vi "Graph_FPGA_stripped_v00.vi"() -> ()   [LabVIEW 2010]
uses:
  Strict Type Defs/Graph Errors.ctl
  Strict Type Defs/Graph Lock Point.ctl
  Strict Type Defs/Graph Output.ctl
  Strict Type Defs/Control Graph Input.ctl
  Strict Type Defs/PII individual.ctl
  Strict Type Defs/Error Scale Graph.ctl
  Strict Type Defs/Lock Thresh Graph.ctl
  Strict Type Defs/Theta graph.ctl
  Strict Type Defs/Safety First.ctl
  Strict Type Defs/Scope.ctl
  Strict Type Defs/Graph Max.ctl
  Strict Type Defs/Graph Min.ctl
  <vilib>/rvi/DataTransferAndStorage/Container/XNode/niFpgaContainer.xnode
  <vilib>/rvi/DataTransferAndStorage/Container/Common/niFpgaContainerMethod.ctl
  <vilib>/rvi/DataTransferAndStorage/Container/Common/niFpgaTransferTypeControl.ctl
  <vilib>/rvi/interface/RandomDataEmulation/nirviRandomDataFPGAFIFO.vi
  <vilib>/rvi/interface/RandomDataEmulation/niFpgaRandomDataHandleErrors.vi
panel:
  out "Min":T1
  out "Max":T2
  in  "Graph Delay(uSec)":u32 caption="Count(uSec)"
  out "HD Errors xp":T3
  in  "Scope":T4={"Trigger Direction"=enum."plus-minus", "Delay"=0, "Aquisition Rate (Ticks)"=40, "Offset"=0, "Channel"=0, "Channel Selector"={"Channel 1"=0, "Channel 2"=4, "Channel 3"=8, "Channel 4"=8}} {"Channel Selector"."Channel 4" items=["Error Signal 1", "Error Signal 2", "Scan Trigger 1", "Scan Trigger 2", "DC Signal 1", "DC Signal 2", "PI Out 1", "PI Out 2"]; "Channel Selector"."Channel 3" items=["Error Signal 1", "Error Signal 2", "Scan Trigger 1", "Scan Trigger 2", "DC Signal 1", "DC Signal 2", "PI Out 1", "PI Out 2"]; "Channel Selector"."Channel 2" items=["Error Signal 1", "Error Signal 2", "Scan Trigger 1", "Scan Trigger 2", "DC Signal 1", "DC Signal 2", "PI Out 1", "PI Out 2"]; "Channel Selector"."Channel 1" items=["Error Signal 1", "Error Signal 2", "Scan Trigger 1", "Scan Trigger 2", "DC Signal 1", "DC Signal 2", "PI Out 1", "PI Out 2"]}
  in  "quit Control Loop":bool
  in  "Control":T5={"PII In 1"={"Lock"=FALSE, "Hold"=FALSE, "P Gain"=0, "P BS"=-5, "I Gain"=0, "I BS"=-10, "I2 G"=0, "I2 BS"=-26, "Scan Amp"=0, "Scan Off"=0, "Scan FS"=0, "SFS BS"=0, "I Max value"=10000, "I2 Max value"=10000, "Scope.Offset"=0, "Trigger Direction"=enum."either", "Scan-PII thresh"=0}, "PII In 2"={"Lock"=FALSE, "Hold"=FALSE, "P Gain"=0, "P BS"=-10, "I Gain"=0, "I BS"=-10, "I2 G"=0, "I2 BS"=-26, "Scan Amp"=0, "Scan Off"=0, "Scan FS"=0, "SFS BS"=0, "I Max value"=10000, "I2 Max value"=10000, "Scope.Offset"=0, "Trigger Direction"=enum."either", "Scan-PII thresh"=0}, "PII In 3"={"Lock"=FALSE, "Hold"=FALSE, "P Gain"=0, "P BS"=-10, "I Gain"=0, "I BS"=-10, "I2 G"=0, "I2 BS"=-26, "Scan Amp"=0, "Scan Off"=0, "Scan FS"=0, "SFS BS"=0, "I Max value"=10000, "I2 Max value"=10000, "Scope.Offset"=0, "Trigger Direction"=enum."either", "Scan-PII thresh"=0}, "PII In 4"={"Lock"=FALSE, "Hold"=FALSE, "P Gain"=0, "P BS"=-10, "I Gain"=0, "I BS"=-10, "I2 G"=0, "I2 BS"=-26, "Scan Amp"=0, "Scan Off"=0, "Scan FS"=0, "SFS BS"=0, "I Max value"=10000, "I2 Max value"=10000, "Scope.Offset"=0, "Trigger Direction"=enum."either", "Scan-PII thresh"=0}, "PII In 5"={"Lock"=FALSE, "Hold"=FALSE, "P Gain"=10, "P BS"=-10, "I Gain"=0, "I BS"=0, "I2 G"=0, "I2 BS"=-26, "Scan Amp"=0, "Scan Off"=0, "Scan FS"=0, "SFS BS"=0, "I Max value"=10000, "I2 Max value"=10000, "Scope.Offset"=0, "Trigger Direction"=enum."either", "Scan-PII thresh"=0}, "PII In 6"={"Lock"=FALSE, "Hold"=FALSE, "P Gain"=0, "P BS"=-10, "I Gain"=0, "I BS"=-10, "I2 G"=0, "I2 BS"=-26, "Scan Amp"=0, "Scan Off"=0, "Scan FS"=0, "SFS BS"=0, "I Max value"=10000, "I2 Max value"=10000, "Scope.Offset"=0, "Trigger Direction"=enum."either", "Scan-PII thresh"=0}, "Error scale"={"Pre-Offset"={"Pre-Offset 1"=2, "Pre-Offset 2"=0, "Pre-Offset 3"=0, "Pre-Offset 4"=0, "Pre-Offset 5"=2, "Pre-Offset 6"=0, "Pre-Offset 7"=0, "Pre-Offset 8"=0}, "Post-Offset "={"Offset 1"=0, "Offset 2"=300, "Offset 3"=0, "Offset 4"=0, "Offset 5"=0, "Offset 6"=0, "Offset 7"=0, "Offset 8"=0}, "Gains"={"Gain 1"=0, "Gain 2"=300, "Gain 3"=0, "Gain 4"=0, "Gain 5"=0, "Gain 6"=0, "Gain 7"=0, "Gain 8"=0}, "Bit Shifts"={"Bit Shift 1"=0, "Bit Shift 2"=300, "Bit Shift 3"=0, "Bit Shift 4"=0, "Bit Shift 5"=0, "Bit Shift 6"=0, "Bit Shift 7"=0, "Bit Shift 8"=0}}, "Lock Thresh"={"Pump A"=0, "Pump B"=0, "EPR"=0, "Graph"=0, "HD A"=40, "HD B"=0}, "Re-Scan Thresh"={"Pump A"=2, "Pump B"=0, "EPR"=40, "Graph"=0, "HD A"=40, "HD B"=0}, "Theta"={"HD A Sin Theta"=0, "HD A Cos Theta"=0, "HD B Sin Theta"=0, "HD B Cos Theta"=0}, "Safety First"={"lim reset"=FALSE, "no limit"=FALSE, "pos slew rate * dt"=10, "neg slew rate * dt"=-10, "Hold All"=FALSE, "Count(Ticks)"=0}}
  in  "\"I too high?\"":T11
  in  "\"Outputs\"":T12
  out "Outputs":T12={"Pump A"=-270, "Pump B"=-1710, "EPR"=880, "Graph"=570, "HD A"=0, "HD B"=0}
  in  "\"Trigger\"":T11
  out "Trigger":T11
  out "Cavity Errors":T13={"Pump A"=0, "Pump B"=1800, "EPR"=0, "Graph"=0, "HD A"=0, "HD B"=0}
  out "Control Loop count":i32=11285327
  out "Scope Full?":bool
  out "Scope loop count":i32=119818
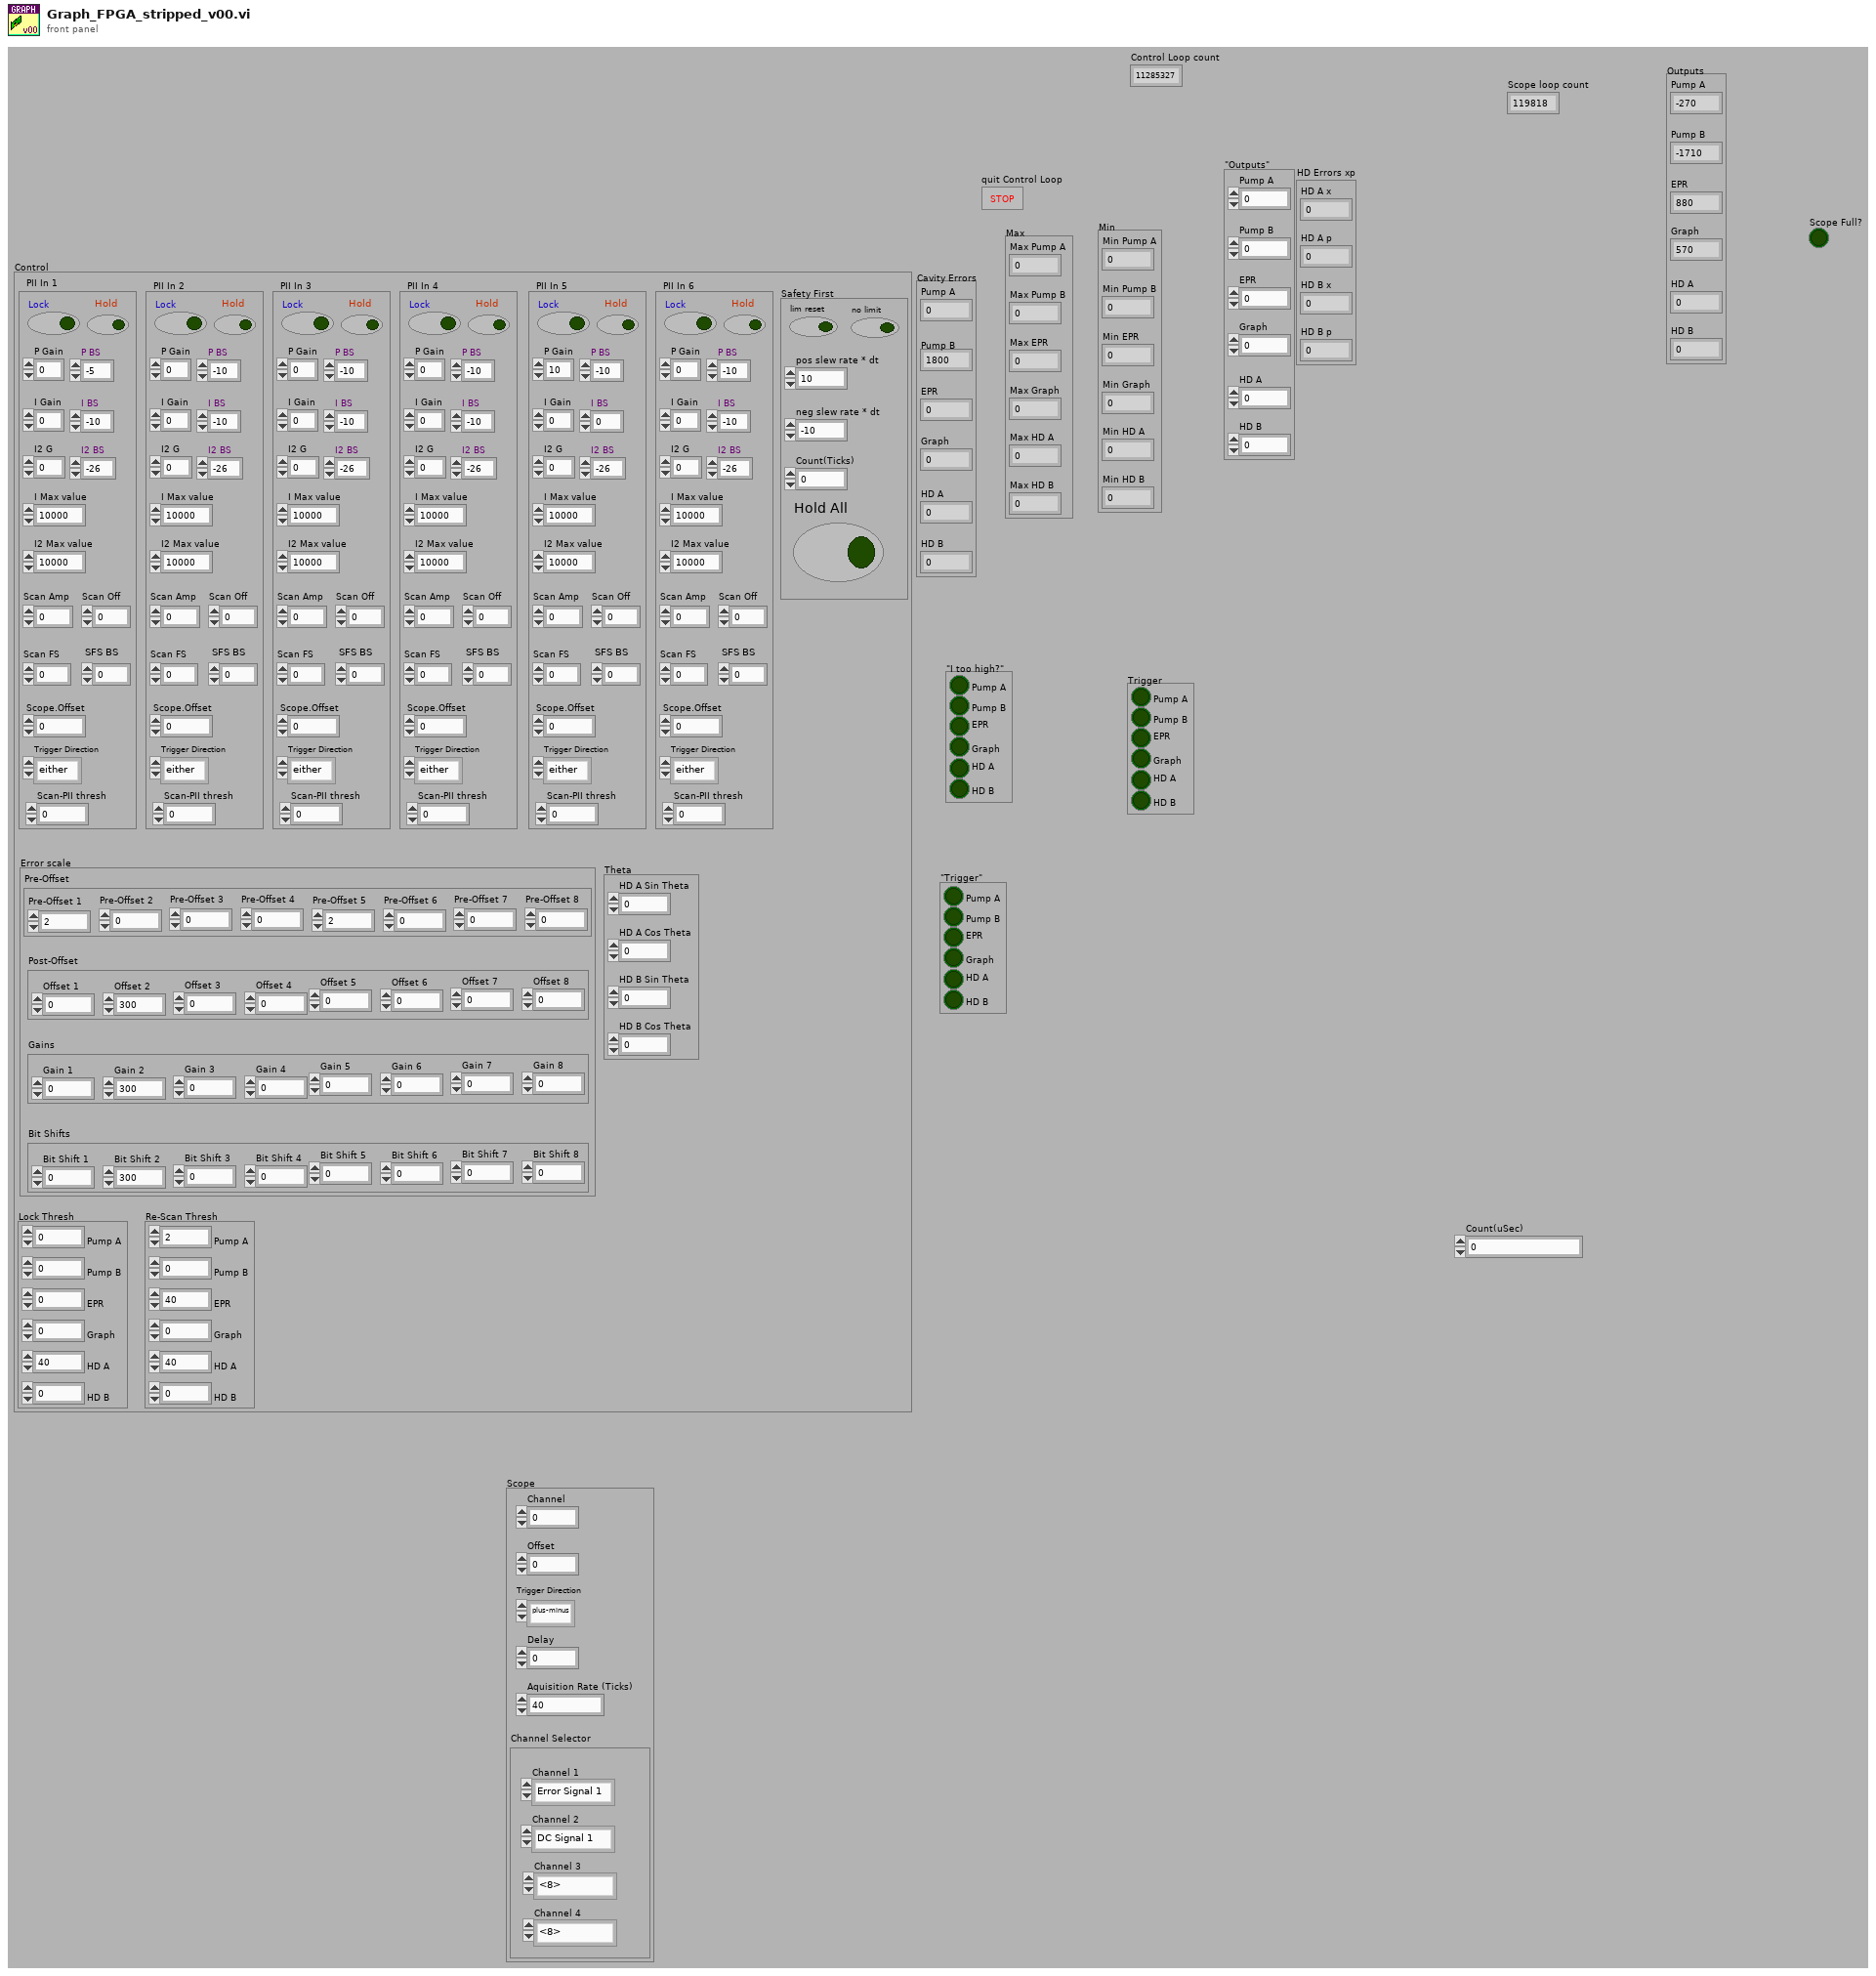
[diagram p1: front panel]
types:
  T1 = typedef "Graph Min.ctl" = cluster{"Min Pump A":i16, "Min Pump B":i16, "Min EPR":i16, "Min Graph":i16, "Min HD A":i16, "Min HD B":i16}
  T2 = typedef "Graph Max.ctl" = cluster{"Max Pump A":i16, "Max Pump B":i16, "Max EPR":i16, "Max Graph":i16, "Max HD A":i16, "Max HD B":i16}
  T3 = cluster{"HD A x":i16, "HD A p":i16, "HD B x":i16, "HD B p":i16}
  T4 = typedef "Scope.ctl" = cluster{"Trigger Direction":enum8{"either", "minus-plus", "plus-minus"}, "Delay":u32, "Aquisition Rate (Ticks)":u32, "Offset":i16, "Channel":i32, "Channel Selector":cluster{"Channel 1":i32, "Channel 2":i32, "Channel 3":i32, "Channel 4":i32}}
  T5 = typedef "Control Graph Input.ctl" = cluster{"PII In 1":T6, "PII In 2":T6, "PII In 3":T6, "PII In 4":T6, "PII In 5":T6, "PII In 6":T6, "Error scale":T7, "Lock Thresh":T8, "Re-Scan Thresh":T8, "Theta":T9, "Safety First":T10}
  T6 = typedef "PII individual.ctl" = cluster{"Lock":bool, "Hold":bool, "P Gain":i32, "P BS":i16, "I Gain":i32, "I BS":i16, "I2 G":i32, "I2 BS":i16, "Scan Amp":i16, "Scan Off":i16, "Scan FS":u16, "SFS BS":i16, "I Max value":i32, "I2 Max value":i32, "Scope.Offset":i16, "Trigger Direction":enum8{"either", "minus-plus", "plus-minus"}, "Scan-PII thresh":i16}
  T7 = typedef "Error Scale Graph.ctl" = cluster{"Pre-Offset":cluster{"Pre-Offset 1":i16, "Pre-Offset 2":i16, "Pre-Offset 3":i16, "Pre-Offset 4":i16, "Pre-Offset 5":i16, "Pre-Offset 6":i16, "Pre-Offset 7":i16, "Pre-Offset 8":i16}, "Post-Offset ":cluster{"Offset 1":i16, "Offset 2":i16, "Offset 3":i16, "Offset 4":i16, "Offset 5":i16, "Offset 6":i16, "Offset 7":i16, "Offset 8":i16}, "Gains":cluster{"Gain 1":i16, "Gain 2":i16, "Gain 3":i16, "Gain 4":i16, "Gain 5":i16, "Gain 6":i16, "Gain 7":i16, "Gain 8":i16}, "Bit Shifts":cluster{"Bit Shift 1":i16, "Bit Shift 2":i16, "Bit Shift 3":i16, "Bit Shift 4":i16, "Bit Shift 5":i16, "Bit Shift 6":i16, "Bit Shift 7":i16, "Bit Shift 8":i16}}
  T8 = typedef "Lock Thresh Graph.ctl" = cluster{"Pump A":i16, "Pump B":i16, "EPR":i16, "Graph":i16, "HD A":i16, "HD B":i16}
  T9 = typedef "Theta graph.ctl" = cluster{"HD A Sin Theta":i32, "HD A Cos Theta":i32, "HD B Sin Theta":i32, "HD B Cos Theta":i32}
  T10 = typedef "Safety First.ctl" = cluster{"lim reset":bool, "no limit":bool, "pos slew rate * dt":i16, "neg slew rate * dt":i16, "Hold All":bool, "Count(Ticks)":u32}
  T11 = typedef "Graph Lock Point.ctl" = cluster{"Pump A":bool, "Pump B":bool, "EPR":bool, "Graph":bool, "HD A":bool, "HD B":bool}
  T12 = typedef "Graph Output.ctl" = cluster{"Pump A":i16, "Pump B":i16, "EPR":i16, "Graph":i16, "HD A":i16, "HD B":i16}
  T13 = typedef "Graph Errors.ctl" = cluster{"Pump A":i16, "Pump B":i16, "EPR":i16, "Graph":i16, "HD A":i16, "HD B":i16}
  T14 = typedef "Signals Graph.ctl" = cluster{"PII In 1":T6, "PII In 2":T6, "PII In 3":T6, "PII In 4":T6, "PII In 5":T6, "PII In 6":T6, "Lock Thresh":T8, "Re-Scan Thresh":T8, "Safety First":T10, "Graph Errors":T13}
  T15 = typedef "Graph Control Cluster.ctl" = cluster{"Control Pump A":T6, "Control Pump B":T6, "Control EPR":T6, "Control Graph":T6, "Control HD A":T6, "Control HD B":T6, "Max":T2, "Min":T1, "Lock Threshold":T8, "Re-Scan Threshold":T8, "Lock Point?":T11, "Re-scan?":T11, "Lock pressed? (-1)":T11, "Cavity Errors":T13, "State (-1)":T16, "Safety First":T10}
  T16 = typedef "Graph State.ctl" = cluster{"Pump A":enum16{"Safe", "Hold", "Scan", "Lock"}, "Pump B":enum16{"Safe", "Hold", "Scan", "Lock"}, "EPR":enum16{"Safe", "Hold", "Scan", "Lock"}, "Graph":enum16{"Safe", "Hold", "Scan", "Lock"}, "HD A":enum16{"Safe", "Hold", "Scan", "Lock"}, "HD B":enum16{"Safe", "Hold", "Scan", "Lock"}}
  T17 = typedef "Graph PII Scan State.ctl" = cluster{"Control Pump A":T6, "Control Pump B":T6, "Control EPR":T6, "Control Graph":T6, "Control HD A":T6, "Control HD B":T6, "Error Signals":T13, "State":T16}
  T18 = typedef "Graph MaxMin.ctl" = cluster{"State":T16, "Reset MaxMin?":T19, "Max":T2, "Min":T1, "Lock pressed?":T11, "Safety First":T10}
  T19 = typedef "Graph Reset MaxMin.ctl" = cluster{"Pump A":bool, "Pump B":bool, "EPR":bool, "Graph":bool, "HD A":bool, "HD B":bool}
  T20 = typedef "niFpgaContainerMethod.ctl" = enum16{"<none>", "write", "read", "clear", "getNumberOfElementsToWrite", "getNumberOfElementsToRead", "enable", "disable", "flushAndDisable", "getStreamState", "readA", "readB", "dramWrite", "dramWriteWithByteEnables", "dramRequestData", "dramRetrieveData"}
  T21 = typedef "niFpgaTransferTypeControl.ctl" = enum16{"Target-Scoped", "Host to Target - DMA", "Target to Host - DMA", "Peer to Peer Reader", "Peer to Peer Writer", "Bidirectional"}
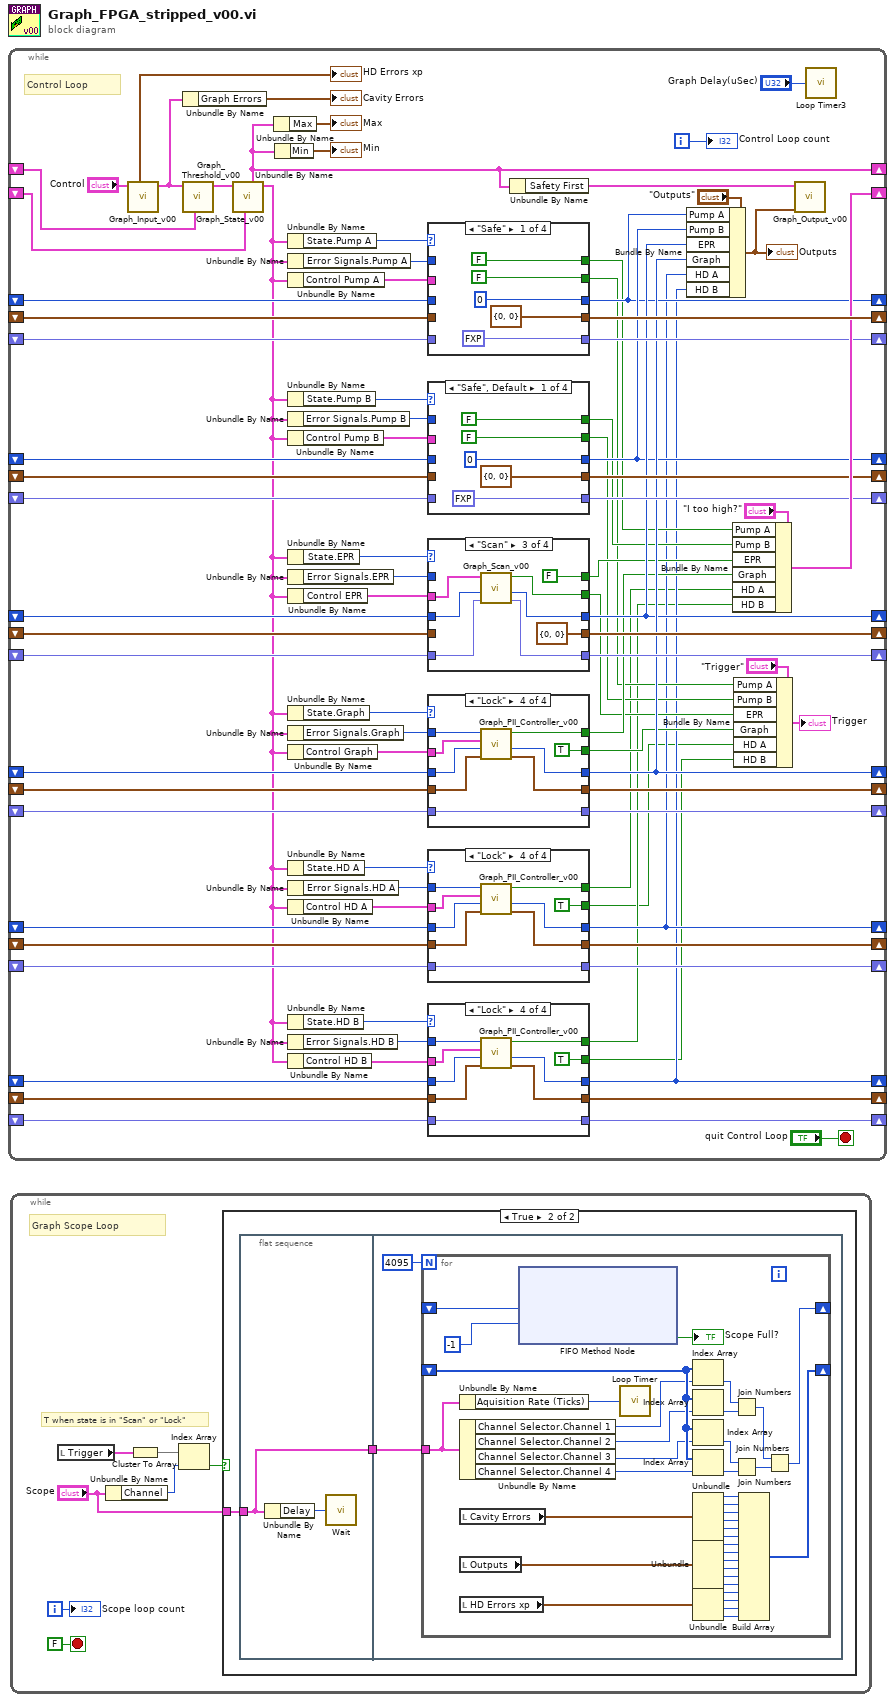
[diagram p0: block diagram]
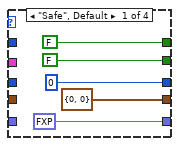
[diagram p3: hidden frame]
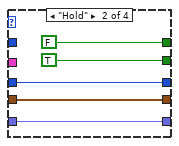
[diagram p4: hidden frame]
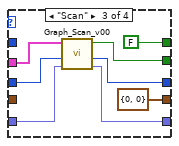
[diagram p5: hidden frame]
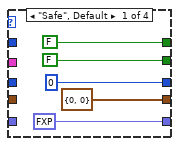
[diagram p6: hidden frame]
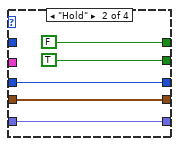
[diagram p7: hidden frame]
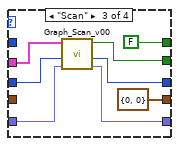
[diagram p8: hidden frame]
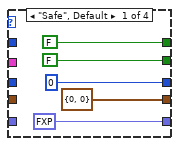
[diagram p9: hidden frame]
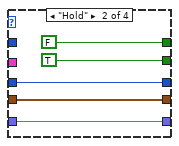
[diagram p10: hidden frame]
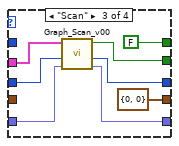
[diagram p11: hidden frame]
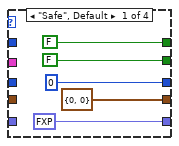
[diagram p12: hidden frame]
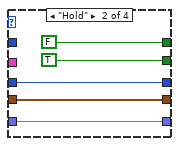
[diagram p13: hidden frame]
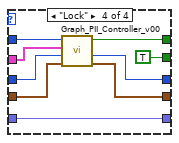
[diagram p14: hidden frame]
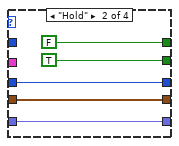
[diagram p15: hidden frame]
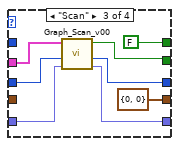
[diagram p16: hidden frame]
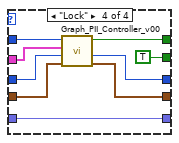
[diagram p17: hidden frame]
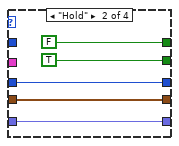
[diagram p18: hidden frame]
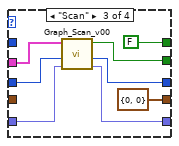
[diagram p19: hidden frame]
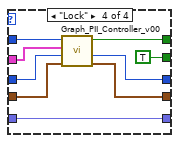
[diagram p20: hidden frame]
diagram:
  n1 = while {
    shift-right: [w86] -> _
    shift-left: _ -> [w84]
    shift-right: [w83] -> _
    shift-left: _ -> [w75]
    shift-right: [w53] -> _
    shift-left: _ -> [w85]
    shift-right: [w80] -> _
    shift-left: _ -> [w79]
    shift-right: [w21] -> _
    shift-left: _ -> [w74]
    shift-right: [w69] -> _
    shift-left: _ -> [w71]
    shift-right: [w54] -> _
    shift-left: _ -> [w70]
    shift-right: [w72] -> _
    shift-left: _ -> [w73]
    shift-right: [w68] -> _
    shift-left: _ -> [w66]
    shift-right: [w55] -> _
    shift-left: _ -> [w67]
    shift-right: [w65] -> _
    shift-left: _ -> [w64]
    shift-right: [w59] -> _
    shift-left: _ -> [w61]
    shift-right: [w56] -> _
    shift-left: _ -> [w60]
    shift-right: [w62] -> _
    shift-left: _ -> [w63]
    shift-right: [w42] -> _
    shift-left: _ -> [w40]
    shift-right: [w32] -> _
    shift-left: _ -> [w41]
    shift-right: [w39] -> _
    shift-left: _ -> [w38]
    shift-right: [w33] -> _
    shift-left: _ -> [w35]
    shift-right: [w31] -> _
    shift-left: _ -> [w34]
    shift-right: [w36] -> _
    shift-left: _ -> [w37]
    i -> [w76]
    stop <- "quit Control Loop" stop-if-true
    # "Control Loop"
    n2 = call "Graph_Input_v00.vi"("Control"="Control") -> ("Signals"=w26:T14, "HD Errors xp"=→"HD Errors xp":T3)  [unwired: 9 in]
    n3 = Unbundle By Name(w26) -> ("Graph Errors"=→"Cavity Errors":T13)
    n4 = call "Graph_Threshold_v00.vi"("MaxMin"=w74, "Signals"=w26) -> ("Control Graph Cluster"=w23:T15)  [unwired: 9 in]
    n5 = call "Graph_State_v00.vi"("\"I too high?\""=w75, "Control Cavity Cluster"=w23) -> ("PII Scan State Errors"=w1:T17, "MaxMin"=w21:T18)  [unwired: 8 in]
    n6 = Unbundle By Name(w21) -> ("Max"=→"Max":T2)
    n7 = Unbundle By Name(w21) -> ("Min"=→"Min":T1)
    n8 = Unbundle By Name(w1) -> ("State.Pump A"=w18:enum16{"Safe", "Hold", "Scan", "Lock"})
    n9 = Unbundle By Name(w1) -> ("Error Signals.Pump A"=w19:i16)
    n10 = Unbundle By Name(w1) -> ("Control Pump A"=w17:T6)
    n11 = Unbundle By Name(w1) -> ("State.Pump B"=w15:enum16{"Safe", "Hold", "Scan", "Lock"})
    n12 = Unbundle By Name(w1) -> ("Error Signals.Pump B"=w16:i16)
    n13 = Unbundle By Name(w1) -> ("Control Pump B"=w14:T6)
    n14 = Unbundle By Name(w1) -> ("State.EPR"=w11:enum16{"Safe", "Hold", "Scan", "Lock"})
    n15 = Unbundle By Name(w1) -> ("Error Signals.EPR"=w12:i16)
    n16 = Unbundle By Name(w1) -> ("Control EPR"=w13:T6)
    n17 = Unbundle By Name(w1) -> ("State.Graph"=w9:enum16{"Safe", "Hold", "Scan", "Lock"})
    n18 = Unbundle By Name(w1) -> ("Error Signals.Graph"=w10:i16)
    n19 = Unbundle By Name(w1) -> ("Control Graph"=w8:T6)
    n20 = Unbundle By Name(w1) -> ("State.HD A"=w7:enum16{"Safe", "Hold", "Scan", "Lock"})
    n21 = Unbundle By Name(w1) -> ("Error Signals.HD A"=w6:i16)
    n22 = Unbundle By Name(w1) -> ("Control HD A"=w5:T6)
    n23 = Unbundle By Name(w1) -> ("State.HD B"=w2:enum16{"Safe", "Hold", "Scan", "Lock"})
    n24 = Unbundle By Name(w1) -> ("Error Signals.HD B"=w4:i16)
    n25 = Unbundle By Name(w1) -> ("Control HD B"=w3:T6)
    n26 = case shown="\"Safe\"" w18 {
      tunnel: w19 -> [_ _ _ w249]
      tunnel: [cluster{"I Cavity":i32, "I2 Cavity":i32} {"I Cavity"=0, "I2 Cavity"=0} ("Integrator") w230 cluster{"I Cavity":i32, "I2 Cavity":i32} {"I Cavity"=0, "I2 Cavity"=0} ("Integrator") w245] -> w86
      tunnel: [FALSE ("I too high? (F=No)") FALSE ("I too high? (F=No)") FALSE ("I too high? (F=No)") w248] -> w52
      tunnel: w17 -> [_ _ w239 w246]
      tunnel: [i16 0 ("PII out") w231 w238 w242] -> w53
      tunnel: w85 -> [_ w231 w235 w243]
      tunnel: w84 -> [_ w230 _ w247]
      tunnel: [fxp<+,33,17> 0.0 ("Scan") w229 w237 w241] -> w80
      tunnel: w79 -> [_ w229 w236 w241]
      tunnel: [FALSE ("Zero Crossing") TRUE ("Zero Crossing") w234 TRUE ("Zero Crossing")] -> w48
      frame "Safe" {
      }
      frame "Hold" {
      }
      frame "Scan" {
        n27 = call "Graph_Scan_v00.vi"("Scan (-1)"=w236, "Scan out (-1)"=w235, "Control Cavity"=w239) -> ("Scan"=w237:fxp<+,33,17>, "Scan out"=w238:i16, "Zero Crossing"=w234:bool)  [unwired: 6 in]
      }
      frame "Lock" {
        n28 = call "Graph_PII_Controller_v00.vi"("Integrator (-1)"=w247, "PII out (-1)"=w243, "Control Cavity"=w246, "OPO A Error"=w249) -> ("Integrator"=w245:cluster{"I Cavity":i32, "I2 Cavity":i32}, "PII out"=w242:i16, "I too high?"=w248:bool)  [unwired: 5 in]
      }
    }
    n29 = case shown="\"Safe\", Default" w15 {
      tunnel: w16 -> [_ _ _ w222]
      tunnel: [cluster{"I Cavity":i32, "I2 Cavity":i32} {"I Cavity"=0, "I2 Cavity"=0} ("Integrator") w203 cluster{"I Cavity":i32, "I2 Cavity":i32} {"I Cavity"=0, "I2 Cavity"=0} ("Integrator") w218] -> w69
      tunnel: [FALSE ("I too high? (F=No)") FALSE ("I too high? (F=No)") FALSE ("I too high? (F=No)") w221] -> w51
      tunnel: w14 -> [_ _ w212 w219]
      tunnel: [i16 0 ("PII out") w204 w211 w216] -> w54
      tunnel: w70 -> [_ w204 w208 w217]
      tunnel: w71 -> [_ w203 _ w220]
      tunnel: [fxp<+,33,17> 0.0 ("Scan") w202 w210 w215] -> w72
      tunnel: w73 -> [_ w202 w209 w215]
      tunnel: [FALSE ("Zero Crossing") TRUE ("Zero Crossing") w206 TRUE ("Zero Crossing")] -> w44
      frame "Safe", Default {
      }
      frame "Hold" {
      }
      frame "Scan" {
        n30 = call "Graph_Scan_v00.vi"("Scan (-1)"=w209, "Scan out (-1)"=w208, "Control Cavity"=w212) -> ("Scan"=w210:fxp<+,33,17>, "Scan out"=w211:i16, "Zero Crossing"=w206:bool)  [unwired: 6 in]
      }
      frame "Lock" {
        n31 = call "Graph_PII_Controller_v00.vi"("Integrator (-1)"=w220, "PII out (-1)"=w217, "Control Cavity"=w219, "OPO A Error"=w222) -> ("Integrator"=w218:cluster{"I Cavity":i32, "I2 Cavity":i32}, "PII out"=w216:i16, "I too high?"=w221:bool)  [unwired: 5 in]
      }
    }
    n32 = case shown="\"Scan\"" w11 {
      tunnel: w12 -> [_ _ _ w195]
      tunnel: [cluster{"I Cavity":i32, "I2 Cavity":i32} {"I Cavity"=0, "I2 Cavity"=0} ("Integrator") w176 cluster{"I Cavity":i32, "I2 Cavity":i32} {"I Cavity"=0, "I2 Cavity"=0} ("Integrator") w191] -> w68
      tunnel: [FALSE ("I too high? (F=No)") FALSE ("I too high? (F=No)") FALSE ("I too high? (F=No)") w194] -> w50
      tunnel: w13 -> [_ _ w185 w192]
      tunnel: [i16 0 ("PII out") w177 w184 w188] -> w55
      tunnel: w67 -> [_ w177 w181 w189]
      tunnel: w66 -> [_ w176 _ w193]
      tunnel: [fxp<+,33,17> 0.0 ("Scan") w175 w183 w187] -> w65
      tunnel: w64 -> [_ w175 w182 w187]
      tunnel: [FALSE ("Zero Crossing") TRUE ("Zero Crossing") w180 TRUE ("Zero Crossing")] -> w47
      frame "Safe", Default {
      }
      frame "Hold" {
      }
      frame "Scan" {
        n33 = call "Graph_Scan_v00.vi"("Scan (-1)"=w182, "Scan out (-1)"=w181, "Control Cavity"=w185) -> ("Scan"=w183:fxp<+,33,17>, "Scan out"=w184:i16, "Zero Crossing"=w180:bool)  [unwired: 6 in]
      }
      frame "Lock" {
        n34 = call "Graph_PII_Controller_v00.vi"("Integrator (-1)"=w193, "PII out (-1)"=w189, "Control Cavity"=w192, "OPO A Error"=w195) -> ("Integrator"=w191:cluster{"I Cavity":i32, "I2 Cavity":i32}, "PII out"=w188:i16, "I too high?"=w194:bool)  [unwired: 5 in]
      }
    }
    n35 = case shown="\"Lock\"" w9 {
      tunnel: w10 -> [_ _ _ w168]
      tunnel: [cluster{"I Cavity":i32, "I2 Cavity":i32} {"I Cavity"=0, "I2 Cavity"=0} ("Integrator") w149 cluster{"I Cavity":i32, "I2 Cavity":i32} {"I Cavity"=0, "I2 Cavity"=0} ("Integrator") w164] -> w59
      tunnel: [FALSE ("I too high? (F=No)") FALSE ("I too high? (F=No)") FALSE ("I too high? (F=No)") w167] -> w49
      tunnel: w8 -> [_ _ w158 w165]
      tunnel: [i16 0 ("PII out") w150 w157 w161] -> w56
      tunnel: w60 -> [_ w150 w154 w162]
      tunnel: w61 -> [_ w149 _ w166]
      tunnel: [fxp<+,33,17> 0.0 ("Scan") w148 w156 w160] -> w62
      tunnel: w63 -> [_ w148 w155 w160]
      tunnel: [FALSE ("Zero Crossing") TRUE ("Zero Crossing") w153 TRUE ("Zero Crossing")] -> w46
      frame "Safe", Default {
      }
      frame "Hold" {
      }
      frame "Scan" {
        n36 = call "Graph_Scan_v00.vi"("Scan (-1)"=w155, "Scan out (-1)"=w154, "Control Cavity"=w158) -> ("Scan"=w156:fxp<+,33,17>, "Scan out"=w157:i16, "Zero Crossing"=w153:bool)  [unwired: 6 in]
      }
      frame "Lock" {
        n37 = call "Graph_PII_Controller_v00.vi"("Integrator (-1)"=w166, "PII out (-1)"=w162, "Control Cavity"=w165, "OPO A Error"=w168) -> ("Integrator"=w164:cluster{"I Cavity":i32, "I2 Cavity":i32}, "PII out"=w161:i16, "I too high?"=w167:bool)  [unwired: 5 in]
      }
    }
    n38 = case shown="\"Lock\"" w7 {
      tunnel: w6 -> [_ _ _ w141]
      tunnel: [cluster{"I Cavity":i32, "I2 Cavity":i32} {"I Cavity"=0, "I2 Cavity"=0} ("Integrator") w122 cluster{"I Cavity":i32, "I2 Cavity":i32} {"I Cavity"=0, "I2 Cavity"=0} ("Integrator") w137] -> w42
      tunnel: [FALSE ("I too high? (F=No)") FALSE ("I too high? (F=No)") FALSE ("I too high? (F=No)") w140] -> w30
      tunnel: w5 -> [_ _ w131 w138]
      tunnel: [i16 0 ("PII out") w123 w130 w134] -> w32
      tunnel: w41 -> [_ w123 w127 w135]
      tunnel: w40 -> [_ w122 _ w139]
      tunnel: [fxp<+,33,17> 0.0 ("Scan") w121 w129 w133] -> w39
      tunnel: w38 -> [_ w121 w128 w133]
      tunnel: [FALSE ("Zero Crossing") TRUE ("Zero Crossing") w126 TRUE ("Zero Crossing")] -> w28
      frame "Safe", Default {
      }
      frame "Hold" {
      }
      frame "Scan" {
        n39 = call "Graph_Scan_v00.vi"("Scan (-1)"=w128, "Scan out (-1)"=w127, "Control Cavity"=w131) -> ("Scan"=w129:fxp<+,33,17>, "Scan out"=w130:i16, "Zero Crossing"=w126:bool)  [unwired: 6 in]
      }
      frame "Lock" {
        n40 = call "Graph_PII_Controller_v00.vi"("Integrator (-1)"=w139, "PII out (-1)"=w135, "Control Cavity"=w138, "OPO A Error"=w141) -> ("Integrator"=w137:cluster{"I Cavity":i32, "I2 Cavity":i32}, "PII out"=w134:i16, "I too high?"=w140:bool)  [unwired: 5 in]
      }
    }
    n41 = case shown="\"Lock\"" w2 {
      tunnel: w4 -> [_ _ _ w114]
      tunnel: [cluster{"I Cavity":i32, "I2 Cavity":i32} {"I Cavity"=0, "I2 Cavity"=0} ("Integrator") w95 cluster{"I Cavity":i32, "I2 Cavity":i32} {"I Cavity"=0, "I2 Cavity"=0} ("Integrator") w110] -> w33
      tunnel: [FALSE ("I too high? (F=No)") FALSE ("I too high? (F=No)") FALSE ("I too high? (F=No)") w113] -> w29
      tunnel: w3 -> [_ _ w104 w111]
      tunnel: [i16 0 ("PII out") w96 w103 w107] -> w31
      tunnel: w34 -> [_ w96 w100 w108]
      tunnel: w35 -> [_ w95 _ w112]
      tunnel: [fxp<+,33,17> 0.0 ("Scan") w94 w102 w106] -> w36
      tunnel: w37 -> [_ w94 w101 w106]
      tunnel: [FALSE ("Zero Crossing") TRUE ("Zero Crossing") w99 TRUE ("Zero Crossing")] -> w27
      frame "Safe", Default {
      }
      frame "Hold" {
      }
      frame "Scan" {
        n42 = call "Graph_Scan_v00.vi"("Scan (-1)"=w101, "Scan out (-1)"=w100, "Control Cavity"=w104) -> ("Scan"=w102:fxp<+,33,17>, "Scan out"=w103:i16, "Zero Crossing"=w99:bool)  [unwired: 6 in]
      }
      frame "Lock" {
        n43 = call "Graph_PII_Controller_v00.vi"("Integrator (-1)"=w112, "PII out (-1)"=w108, "Control Cavity"=w111, "OPO A Error"=w114) -> ("Integrator"=w110:cluster{"I Cavity":i32, "I2 Cavity":i32}, "PII out"=w107:i16, "I too high?"=w113:bool)  [unwired: 5 in]
      }
    }
    n44 = Unbundle By Name(w21) -> ("Safety First"=w58:T10)
    n45 = Bundle By Name(cluster="\"Outputs\"", "Pump A"=w53, "Pump B"=w54, "EPR"=w55, "Graph"=w56, "HD A"=w32, "HD B"=w31) -> (w57:T12)
    "Outputs" <- w57
    n46 = Bundle By Name(cluster="\"I too high?\"", "Pump A"=w52, "Pump B"=w51, "EPR"=w50, "Graph"=w49, "HD A"=w30, "HD B"=w29) -> (w83:T11)
    n47 = Bundle By Name(cluster="\"Trigger\"", "Pump A"=w48, "Pump B"=w44, "EPR"=w47, "Graph"=w46, "HD A"=w28, "HD B"=w27) -> (→"Trigger":T11)
    n48 = call "Graph_Output_v00.vi"("Outputs"=w57, "Safety First"=w58) -> ()  [unwired: 10 in]
    n49 = call "Loop Timer3"("Count(uSec)"="Graph Delay(uSec)") -> ()  [unwired: 1 out]
    "Control Loop count" <- w76
  }
  n50 = while {
    i -> [w253]
    stop <- FALSE ("stop") stop-if-true
    # "Graph Scope Loop"
    # "T when state is in \"Scan\" or \"Lock\""
    n51 = local read "Trigger"() -> (w251:T11)
    n52 = Unbundle By Name("Scope") -> ("Channel"=w254:i32)
    n53 = Cluster To Array(cluster=w251) -> (array=w255:bool[])
    n54 = Index Array(array=w255, index=w254) -> (element=w252:bool)
    n55 = case shown="True" w252 {
      tunnel: "Scope" -> [_ w258]
      frame False {
      }
      frame True {
        n56 = flat-sequence {
          tunnel: w258 -> [w259]
          tunnel: [w259] -> w257
          tunnel: w257 -> [w261]
          frame #0 {
            n57 = Unbundle By Name(w259) -> ("Delay"=w260:u32)
            n58 = call "Wait"("Count(Ticks)"=w260) -> ()  [unwired: 1 out]
          }
          frame #1 {
            n59 = for {
              N: 4095 -> [_]
              tunnel: w261 -> [w298]
              shift-right: [w290] -> _
              shift-left: _ -> [w289]
              shift-right: [w285] -> _
              shift-left: _ -> [w284]
              n60 = Unbundle By Name(w298) -> ("Aquisition Rate (Ticks)"=w299:u32)
              n61 = Unbundle By Name(w298) -> ("Channel Selector.Channel 1"=w286:i32, "Channel Selector.Channel 2"=w287:i32, "Channel Selector.Channel 3"=w281:i32, "Channel Selector.Channel 4"=w288:i32)
              n62 = local read "Cavity Errors"() -> (w297:T13)
              n63 = local read "Outputs"() -> (w296:T12)
              n64 = local read "HD Errors xp"() -> (w279:T3)
              n65 = xnode ("FIFO Method Node")("Element"=w284, "Timeout"=-1) -> ("Timed Out?"=→"Scope Full?":bool)  [unwired: 1 in, 1 out]
              n66 = call "Loop Timer"("Count(uSec)"=w299) -> ()  [unwired: 1 out]
              n67 = Index Array(array=w289, index=w286) -> (element=w292:i16)
              n68 = Index Array(array=w289, index=w287) -> (element=w291:i16)
              n69 = Index Array(array=w289, index=w281) -> (element=w280:i16)
              n70 = Index Array(array=w289, index=w288) -> (element=w293:i16)
              n71 = Unbundle(w297) -> ("Pump A"=w278:i16, "Pump B"=w277:i16, "EPR"=w276:i16, "Graph"=w275:i16, "HD A"=w274:i16, "HD B"=w273:i16)
              n72 = Unbundle(w296) -> ("Pump A"=w272:i16, "Pump B"=w271:i16, "EPR"=w270:i16, "Graph"=w269:i16, "HD A"=w268:i16, "HD B"=w267:i16)
              n73 = Unbundle(w279) -> ("HD A x"=w266:i16, "HD A p"=w265:i16, "HD B x"=w264:i16, "HD B p"=w263:i16)
              n74 = Join Numbers(hi=w292, lo=w291) -> ((hi.lo)=w295:u32)
              n75 = Join Numbers(hi=w280, lo=w293) -> ((hi.lo)=w294:u32)
              n76 = Build Array(w278, w277, w276, w275, w274, w273, w272, w271, w270, w269, w268, w267, w266, w265, w264, w263) -> (w290:i16[])
              n77 = Join Numbers(hi=w295, lo=w294) -> ((hi.lo)=w285:u64)
            }
          }
        }
      }
    }
    "Scope loop count" <- w253
  }
